vi "XY Graph Save Selected Plots Event.vi"(6 "Delimiter (TAB)":string="\t", 7 "X Axis Option (Dialog)":T1(ring), 8 "Error In":errorcluster, 9 "Save All Plots? (T)":bool=TRUE, 10 "File Path in":path, 11 "XYGraph Ref":T2) -> (0 "Error Out":errorcluster, 1 "Message":string, 2 "File Path out":path, 3 "Saved Plot Names":string[](array[string]), 4 "Saved Plot Indices":i32[](array[numeric]), 5 "Graph Name":string)   [LabVIEW 2019, in "XY Graph Add-Ons.lvlib"]
uses:
  XY Graph Add-Ons.lvlib
  XY Graph Refnum.ctl
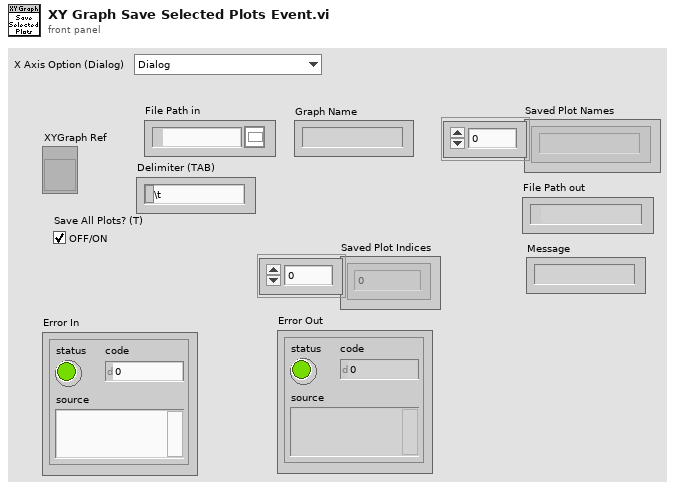
[diagram p1: front panel]
types:
  T1 = enum16{"Dialog", "Save Single X Axis if Common", "Save X Axis for each Plot"}
  T2 = typedef "XY Graph Add-Ons.lvlib/XY Graph Refnum.ctl" = refnum<vi>
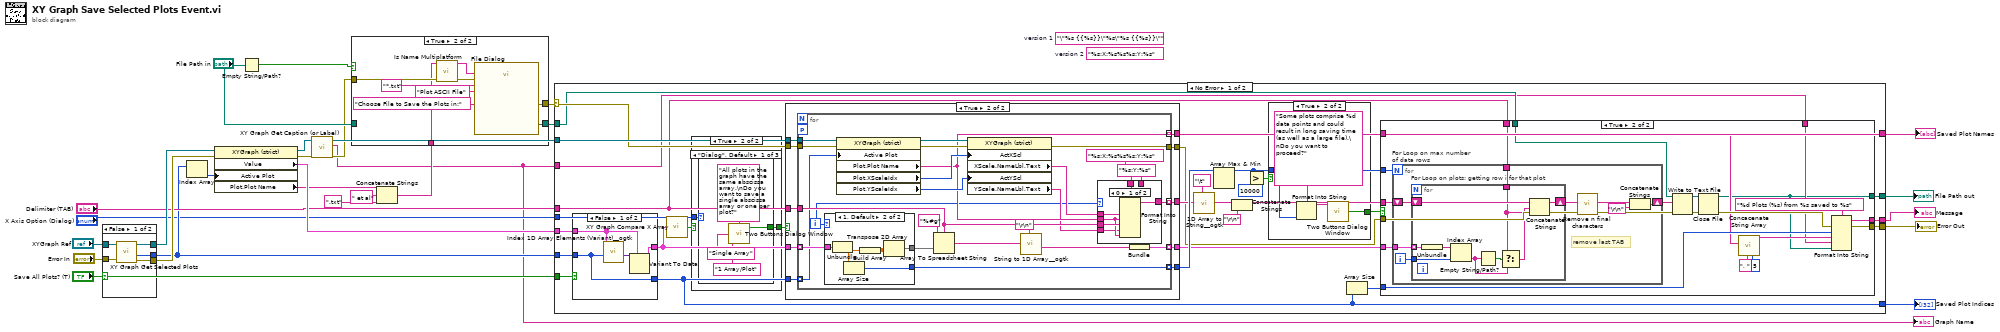
[diagram p0: block diagram]
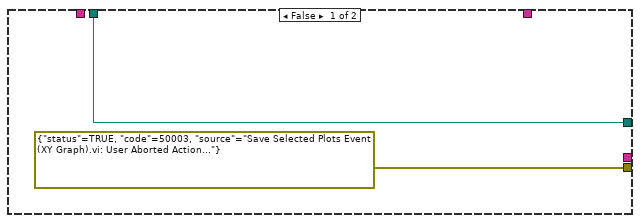
[diagram p4: hidden frame]
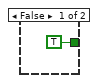
[diagram p5: hidden frame]
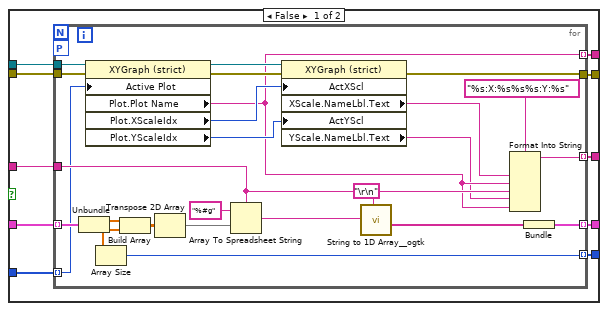
[diagram p6: hidden frame]
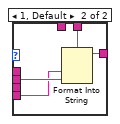
[diagram p7: hidden frame]
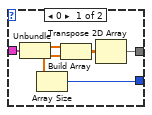
[diagram p8: hidden frame]
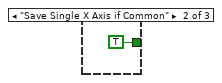
[diagram p10: hidden frame]
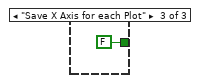
[diagram p11: hidden frame]
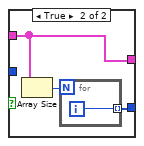
[diagram p12: hidden frame]
diagram:
  (unwired) "%s:X:%s%s%s:Y:%s"  # version 2
  (unwired) "\"%s {{%s}}\"%s\"%s {{%s}}\""  # version 1
  n1 = case shown="False" "Save All Plots? (T)" {
    tunnel: "XYGraph Ref" -> [w33 w35]
    tunnel: "Error In" -> [w32 w34]
    tunnel: [w31 w35] -> w26
    tunnel: [w30 _] -> w14
    tunnel: [w29 w34] -> w21
    frame False {
      n2 = call "XY Graph Get Selected Plots.vi"("error in (no error)"=w32, "XYGraph in"=w33) -> ("error out"=w29:errorcluster, "Selected Plots"=w30:i32[], "XYGraph out"=w31:T2)  [unwired: 5 in, 2 out]
    }
    frame True {
    }
  }
  n3 = Index Array(array=w14) -> (element=w13:i32)  [unwired: 1 in]
  n4 = property class="XYGraph (strict)"(reference=w26, error in=w21, "Active Plot"=w13) -> (reference out=w24:T2, error out=w3:errorcluster, "Value"=w25:cluster{"X Array":dbl[], "Y Array":dbl[]}[], "Plot.Plot Name"=w12:string)
  n5 = Empty String/Path?(string/path="File Path in") -> (empty?=w8:bool)
  n6 = call "XY Graph Get Caption (or Label).vi"("error in (no error)"=w3, "XYGraph in"=w24) -> ("error out"=w2:errorcluster, "Caption (or Label) Text"=w1:string, "XYGraph out"=w4:T2)  [unwired: 7 in]
  "Graph Name" <- w1
  n7 = Concatenate Strings(w12, " et al" ("string"), ".txt" ("string")) -> (w9:string)
  n8 = case shown="True" w8 {
    tunnel: [w36 w43] -> w20
    tunnel: [w37 w42] -> w19
    tunnel: w2 -> [w36 w41]
    tunnel: w9 -> [_ w38]
    tunnel: "File Path in" -> [w37 _]
    frame False {
    }
    frame True {
      n9 = call <vilib>:"Is Name Multiplatform.vi"("error in (no error)"=w41, "filename"=w38) -> ("error out"=w40:errorcluster, "suggested filename"=w39:string)  [unwired: 5 in, 3 out]
      n10 = call "File Dialog"("prompt"="Choose File to Save the Plots in:", "default name"=w39, "error in"=w40, "pattern (all files)"="*.txt", "pattern label"="Plot ASCII File") -> ("selected path"=w42:path, "error out"=w43:errorcluster)  [unwired: 7 in, 2 out]
    }
  }
  n11 = case shown="No Error" w20 {
    selector: w20 -> [w72 w228]
    tunnel: w25 -> [w76 _]
    tunnel: w4 -> [w75 _]
    tunnel: [w48 _] -> w23
    tunnel: [w53 w228] -> w22
    tunnel: w14 -> [w65 _]
    tunnel: w19 -> [w54 _]
    tunnel: [w52 _] -> w18
    tunnel: "Save All Plots? (T)" -> [w66 _]
    tunnel: [w51 _] -> w16
    tunnel: "Delimiter (TAB)" -> [w64 _]
    tunnel: "X Axis Option (Dialog)" -> [w60 _]
    tunnel: [w49 _] -> w5
    tunnel: w1 -> [w47 _]
    frame No Error {
      n12 = case shown="False" w66 {
        tunnel: w76 -> [w222 w226]
        tunnel: [w221 w226] -> w63
        tunnel: w65 -> [w220 _]
        tunnel: [w220 w224] -> w51
        frame False {
          n13 = call <userlib>:"Index 1D Array Elements (Variant)__ogtk.vi"("indices"=w220, "array"=w222) -> ("elements"=w223:variant[])  [unwired: 9 in]
          n14 = Variant To Data(type=w222, Variant=w223) -> (data=w221:cluster{"X Array":dbl[], "Y Array":dbl[]}[])  [unwired: 1 in, 1 out]
        }
        frame True {
          n15 = Array Size(array=w226) -> (size(s)=w225:i32)
          n16 = for {
            N: w225 -> [_]
            tunnel: [w227] -> w224 mode=indexing
            i -> [w227]
          }
        }
      }
      n17 = call "XY Graph Compare X Array.vi"("Plot Array"=w63) -> ("Same [X]?"=w62:bool)  [unwired: 8 in]
      n18 = case shown="True" w62 {
        selector: w62 -> [w211 _]
        tunnel: [w211 w213] -> w61
        tunnel: w60 -> [_ w212]
        frame False {
        }
        frame True {
          n19 = case shown="\"Dialog\", Default" w212 {
            tunnel: [w214 TRUE ("T button?") FALSE ("T button?")] -> w213
            frame "Dialog", Default {
              n20 = call "Two Buttons Dialog Window.vi"("Cancel Button Text"="1 Array/Plot" ("F button name (\"Cancel\")"), "OK Button Text"="Single Array" ("T button name (\"OK\")"), "Message"="All plots in the graph have the same abscissa array.\nDo you want to save a single abscissa array or one per plot?" ("message")) -> ("OK?"=w214:bool)
            }
            frame "Save Single X Axis if Common" {
            }
            frame "Save X Axis for each Plot" {
            }
          }
        }
      }
      n21 = case shown="True" w61 {
        tunnel: w75 -> [w130 w165]
        tunnel: [w129 w164] -> w48
        tunnel: [w128 w163] -> w74
        tunnel: [w127 w162] -> w73
        tunnel: w72 -> [w126 w161]
        tunnel: [w125 w160] -> w71
        tunnel: [w124 w159] -> w55
        tunnel: w64 -> [w123 w158]
        tunnel: w51 -> [w122 w157]
        tunnel: w63 -> [w121 w156]
        frame False {
          n22 = for {
            tunnel: w121 -> [w155] mode=indexing
            tunnel: w130 -> [w154]
            tunnel: [w134] -> w129 mode=indexing
            tunnel: w126 -> [w153]
            tunnel: [w146] -> w124
            tunnel: [w136] -> w127 mode=indexing
            tunnel: [w140] -> w128 mode=indexing
            tunnel: [w142] -> w125 mode=indexing
            workers-P: _ -> [_]
            tunnel: w123 -> [w135]
            tunnel: w122 -> [w131] mode=indexing
            n23 = Unbundle(w155) -> ("X Array"=w148:dbl[], "Y Array"=w141:dbl[])
            n24 = property class="XYGraph (strict)"(reference=w154, error in=w153, "Active Plot"=w131) -> (reference out=w152:T2, error out=w147:errorcluster, "Plot.Plot Name"=w134:string, "Plot.XScaleIdx"=w145:u32, "Plot.YScaleIdx"=w144:u32)
            n25 = Array Size(array=w141) -> (size(s)=w140:i32)
            n26 = Build Array(w148, w141) -> (w151:dbl[][])
            n27 = Transpose 2D Array(2D array=w151) -> (transposed array=w150:dbl[][])
            n28 = Array To Spreadsheet String(delimiter (Tab)=w135, array=w150, 3:"%#g" ("format string")) -> (spreadsheet string=w138:string)
            n29 = property class="XYGraph (strict)"(reference=w152, error in=w147, "ActXScl"=w145, "ActYScl"=w144) -> (error out=w146:errorcluster, "XScale.NameLbl.Text"=w133:string, "YScale.NameLbl.Text"=w132:string)  [unwired: 1 out]
            n30 = call <userlib>:"String to 1D Array__ogtk.vi"("delimiter (Tab)"="\r\n", "string"=w138) -> ("Array of Strings"=w137:string[])  [unwired: 9 in]
            n31 = Format Into String(format string="%s:X:%s%s%s:Y:%s", w133, w134, w135, w132, w134) -> (resulting string=w142:string)  [unwired: 2 in, 1 out]
            n32 = Bundle("Array of Strings"=w137) -> (w136:cluster{"Array of Strings":string[]})  [unwired: 1 in]
          }
        }
        frame True {
          n33 = for {
            tunnel: w156 -> [w189] mode=indexing
            tunnel: w165 -> [w188]
            tunnel: [w171] -> w164 mode=indexing
            tunnel: w161 -> [w187]
            tunnel: [w182] -> w159
            tunnel: [w173] -> w162 mode=indexing
            tunnel: [w177] -> w163 mode=indexing
            tunnel: [w178] -> w160 mode=indexing
            workers-P: _ -> [_]
            tunnel: w158 -> [w172]
            tunnel: w157 -> [w168] mode=indexing
            i -> [w167]
            n34 = case shown="1, Default" w167 {
              tunnel: w189 -> [w205 w210]
              tunnel: [w203 w208] -> w185
              tunnel: [w200 w206] -> w177
              frame 0 {
                n35 = Unbundle(w205) -> ("X Array"=w202:dbl[], "Y Array"=w201:dbl[])
                n36 = Array Size(array=w201) -> (size(s)=w200:i32)
                n37 = Build Array(w202, w201) -> (w204:dbl[][])
                n38 = Transpose 2D Array(2D array=w204) -> (transposed array=w203:dbl[][])
              }
              frame 1, Default {
                n39 = Unbundle(w210) -> ("Y Array"=w207:dbl[])  [unwired: 1 out]
                n40 = Array Size(array=w207) -> (size(s)=w206:i32)
                n41 = Build Array(w207) -> (w209:dbl[][])
                n42 = Transpose 2D Array(2D array=w209) -> (transposed array=w208:dbl[][])
              }
            }
            n43 = property class="XYGraph (strict)"(reference=w188, error in=w187, "Active Plot"=w168) -> (reference out=w186:T2, error out=w183:errorcluster, "Plot.Plot Name"=w171:string, "Plot.XScaleIdx"=w181:u32, "Plot.YScaleIdx"=w180:u32)
            n44 = Array To Spreadsheet String(delimiter (Tab)=w172, array=w185, 3:"%#g" ("format string")) -> (spreadsheet string=w175:string)
            n45 = property class="XYGraph (strict)"(reference=w186, error in=w183, "ActXScl"=w181, "ActYScl"=w180) -> (error out=w182:errorcluster, "XScale.NameLbl.Text"=w170:string, "YScale.NameLbl.Text"=w169:string)  [unwired: 1 out]
            n46 = call <userlib>:"String to 1D Array__ogtk.vi"("delimiter (Tab)"="\r\n", "string"=w175) -> ("Array of Strings"=w174:string[])  [unwired: 9 in]
            n47 = case shown="0" w167 {
              tunnel: "%s:X:%s%s%s:Y:%s" ("format string") -> [w195 _]
              tunnel: [w194 w199] -> w178
              tunnel: w172 -> [w193 _]
              tunnel: w171 -> [w192 w198]
              tunnel: w170 -> [w191 _]
              tunnel: w169 -> [w190 w197]
              tunnel: "%s:Y:%s" ("format string") -> [_ w196]
              frame 0 {
                n48 = Format Into String(format string=w195, w191, w192, w193, w190, w192) -> (resulting string=w194:string)  [unwired: 2 in, 1 out]
              }
              frame 1, Default {
                n49 = Format Into String(format string=w196, w197, w198) -> (resulting string=w199:string)  [unwired: 2 in, 1 out]
              }
            }
            n50 = Bundle("Array of Strings"=w174) -> (w173:cluster{"Array of Strings":string[]})  [unwired: 1 in]
          }
        }
      }
      n51 = call <userlib>:"1D Array to String__ogtk.vi"("delimiter (Tab)"="\t", "Array of Strings"=w71) -> ("delimited string"=w69:string)  [unwired: 9 in]
      n52 = Array Max & Min(array=w74) -> (max value=w57:i32)  [unwired: 3 out]
      n53 = Concatenate Strings(w69, "\r\n") -> (w68:string)
      n54 = Greater?(x=w57, y=10000) -> (0:w58:bool)
      n55 = case shown="True" w58 {
        tunnel: [TRUE ("T button?") w118] -> w56
        tunnel: w57 -> [_ w117]
        frame False {
        }
        frame True {
          n56 = Format Into String(format string="Some plots comprise %d data points and could result in long saving time (as well as a large file).\nDo you want to proceed?", w117) -> (resulting string=w119:string)  [unwired: 2 in, 1 out]
          n57 = call "Two Buttons Dialog Window.vi"("Message"=w119) -> ("OK?"=w118:bool)  [unwired: 2 in]
        }
      }
      n58 = Array Size(array=w51) -> (size(s)=w50:i32)
      n59 = case shown="True" w56 {
        tunnel: w73 -> [_ w98]
        tunnel: w68 -> [_ w97]
        tunnel: w64 -> [_ w96]
        tunnel: w57 -> [_ w95]
        tunnel: w55 -> [_ w94]
        tunnel: w54 -> [w78 w92]
        tunnel: [errorcluster {"status"=TRUE, "code"=50003, "source"="Save Selected Plots Event (XY Graph).vi: User Aborted Action..."} ("error IO") w85] -> w53
        tunnel: [w78 w79] -> w52
        tunnel: w50 -> [_ w84]
        tunnel: [_ w82] -> w49
        tunnel: w48 -> [_ w81]
        tunnel: w47 -> [_ w80]
        frame False {
        }
        frame True {
          n60 = for "For Loop on max number of data rows" {
            N: w95 -> [_]
            tunnel: w98 -> [w106]
            shift-right: [w102] -> w93
            shift-left: w97 -> [w105]
            tunnel: w96 -> [w99]
            i -> [w104]
            # "remove last TAB"
            n61 = for "For Loop on plots: getting row i for that plot" {
              tunnel: w106 -> [w115] mode=indexing
              shift-right: [w108] -> w103
              shift-left: w105 -> [w110]
              tunnel: w104 -> [w113]
              tunnel: w99 -> [w107]
              n62 = Unbundle(w115) -> ("Array of Strings"=w114:string[])
              n63 = Index Array(array=w114, index=w113) -> (element=w111:string)
              n64 = Empty String/Path?(string/path=w111) -> (empty?=w112:bool)
              n65 = Select(t=w107, s=w112, f=w111) -> (s? t:f=w109:string)
              n66 = Concatenate Strings(w110, w109, w107) -> (w108:string)
            }
            n67 = call "Remove n final characters.vi"("String in"=w103) -> ("String out"=w100:string)  [unwired: 8 in]
            n68 = Concatenate Strings(w100, "\r\n") -> (w102:string)
          }
          n69 = Write to Text File(file (use dialog)=w92, text=w93, error in=w94) -> (refnum out=w90:refnum<file>, error out=w91:errorcluster)  [unwired: 1 in, 1 out]
          n70 = Close File(refnum=w90, error in=w91) -> (path=w79:path, error out=w86:errorcluster)
          n71 = call "Concacenate String Array.vi"("Max Number of Elements (None: -1)"=5 ("Max Number of Elements (None: 1)"), "Separator (TAB)"=", ", "String Array"=w81) -> ("Formatted String"=w87:string)  [unwired: 8 in]
          n72 = Format Into String(format string="%d Plots (%s) from %s saved to %s", error in=w86, w84, w87, w80, w79) -> (resulting string=w82:string, error out=w85:errorcluster)  [unwired: 1 in]
        }
      }
    }
    frame Error {
    }
  }
  "Error Out" <- w22
  "Saved Plot Indices" <- w16
  "Saved Plot Names" <- w23
  "File Path out" <- w18
  "Message" <- w5
